vi "CheckResponce.vi"(11 "Responce":u8[](array[numeric])=[2, 48, 49, 65, 77, 73, 44, 79, 75, 44, 84, 69, 77, 80, 45, 50, 48, 48, 48, 32, 32, 86, 48, 48, 45, 82, 48, 48, 50, 52, 13, 10] format="%x") -> (3 "Error Code":i8)   [LabVIEW 2017]
uses:
  <instrlib>/Samwontech TEMP2xxx/Samwontech TEMP2xxx.lvlib
panel:
  in  "Error Responce":u8[](array[numeric])=[2, 48, 49, 78, 71, 48, 49, 53, 55, 13, 10] format="%x"
  out "Responce":string
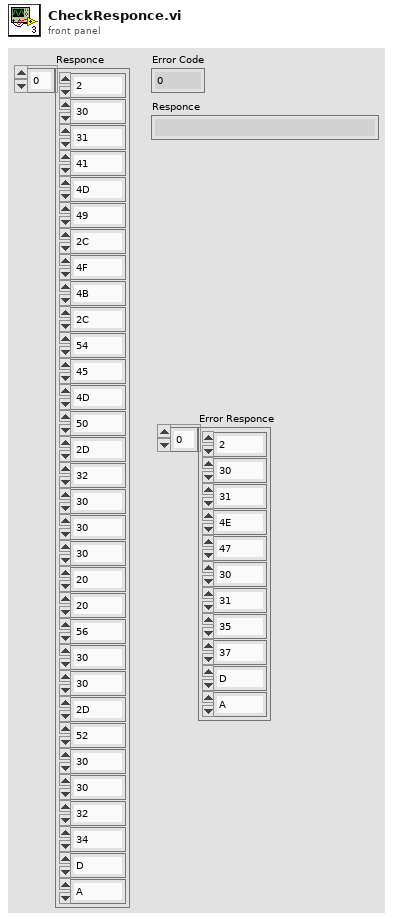
[diagram p1: front panel]
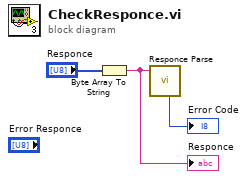
[diagram p0: block diagram]
diagram:
  n1 = Byte Array To String(unsigned byte array="Responce") -> (string=w3:string)
  "Responce" <- w3
  n2 = call <instrlib>:"Responce Parse.vi"("Responce"=w3) -> ("Error Code"=→"Error Code":i8)  [unwired: 4 in, 6 out]
